vi "CaseStatement1.vi"() -> ()   [LabVIEW 2014]
panel:
  in  "Subtract":bool
  in  "Multiply":bool
  in  "Add":bool
  out "Result":dbl
  in  "B":dbl
  in  "A":dbl
  out "Multiplied":bool
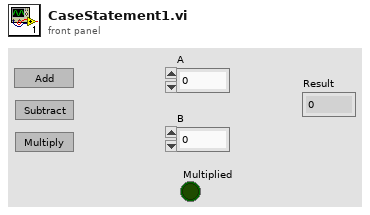
[diagram p1: front panel]
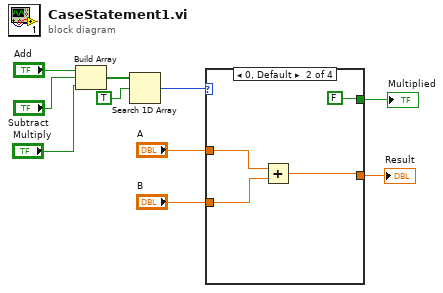
[diagram p0: block diagram]
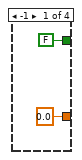
[diagram p2: hidden frame]
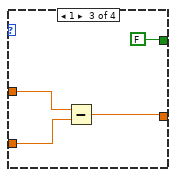
[diagram p3: hidden frame]
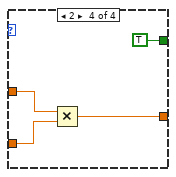
[diagram p4: hidden frame]
diagram:
  n1 = Build Array("Add", "Subtract", "Multiply") -> (w3:bool[])
  n2 = Search 1D Array(1D array=w3, element=TRUE) -> (index of element=w1:i32)  [unwired: 1 in]
  n3 = case shown="0, Default" w1 {
    tunnel: "A" -> [_ w16 w20 w24]
    tunnel: "B" -> [_ w15 w19 w23]
    tunnel: [0.0 w14 w18 w22] -> w8
    tunnel: [FALSE FALSE FALSE TRUE] -> w7
    frame -1 {
    }
    frame 0, Default {
      n4 = Add(x=w16, y=w15) -> (x+y=w14:dbl)
    }
    frame 1 {
      n5 = Subtract(x=w20, y=w19) -> (x-y=w18:dbl)
    }
    frame 2 {
      n6 = Multiply(x=w24, y=w23) -> (x*y=w22:dbl)
    }
  }
  "Multiplied" <- w7
  "Result" <- w8
